vi "First Test.vi"() -> ()   [LabVIEW 2013]
uses:
  source/JKI SM/JKI SM.lvclass
panel:
  out "Macro String":string
  in  "Category":string="UI"
  out "All State Frames":string[](array[string])
  out "State Frames":string[](array[string])
  out "error out 2":errorcluster
  out "Is a JKI State Machine 2":bool
  out "Is a JKI State Machine":bool
  out "error out":errorcluster
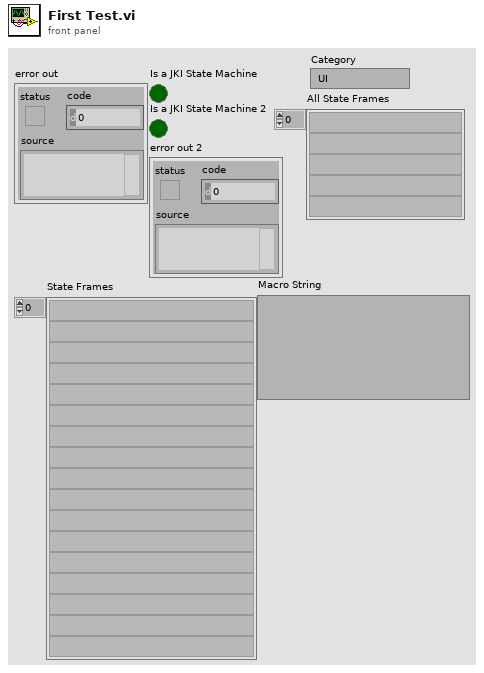
[diagram p1: front panel]
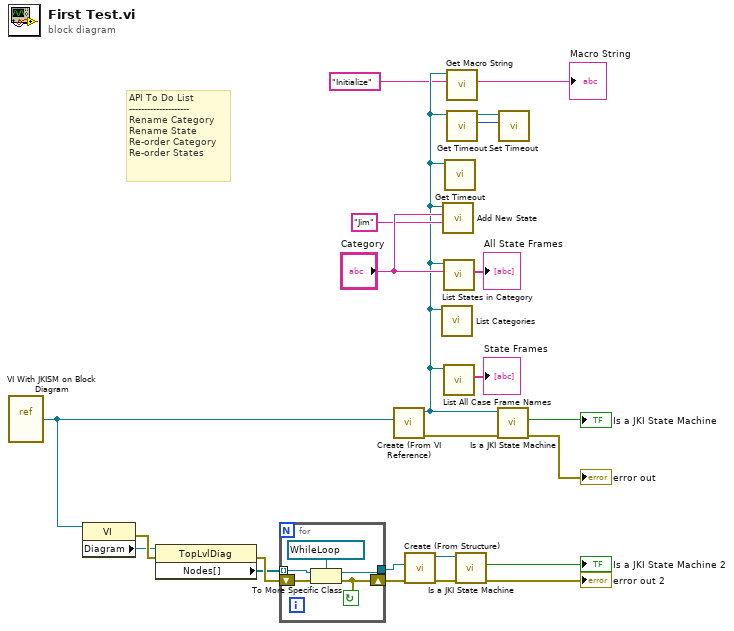
[diagram p0: block diagram]
diagram:
  # "API To Do List\n--------------------\nRename Category\nRename State\nRe-order Category\nRe-order States"
  n1 = vi-ref "VI With JKISM on Block Diagram.vi"() -> (w16:refnum<vi>)
  n2 = property class="VI"(reference=w16) -> (error out=w20:errorcluster, "Diagram"=w17:refnum<vi>)  [unwired: 1 in, 1 out]
  n3 = property class="TopLvlDiag"(reference=w17, error in=w20) -> (error out=w19:errorcluster, "Nodes[]"=w18:refnum<vi>[])  [unwired: 1 out]
  n4 = for {
    tunnel: w18 -> [w27] mode=indexing
    tunnel: [w25] -> w14
    shift-right: [w24] -> w15
    shift-left: w19 -> [w26]
    stop <- w24 continue-if-true
    n5 = To More Specific Class(target class=refnum<vi> refnum ("WLoop Refnum"), reference=w27, error in=w26) -> (specific class reference=w25:refnum<vi>, error out=w24:errorcluster)
  }
  n6 = call "Create (From VI Reference).vi"("VI"=w16) -> ("error out"=w23:errorcluster, "JKI SM out"=w3:refnum<class "JKI SM.lvclass">)  [unwired: 9 in]
  n7 = call "Create (From Structure).vi"("error in (no error)"=w15, "Structure"=w14) -> ("error out"=w13:errorcluster, "JKI SM out"=w12:refnum<class "JKI SM.lvclass">)  [unwired: 8 in]
  n8 = call "List Categories.vi"("JKI SM in"=w3) -> ()  [unwired: 7 in, 4 out]
  n9 = call "Add New State.vi"("State Name"="Jim", "Category (Optional)"="Category", "JKI SM in"=w3) -> ()  [unwired: 7 in, 2 out]
  n10 = call "List States in Category.vi"("Category"="Category", "JKI SM in"=w3) -> ("States"=→"All State Frames":string[])  [unwired: 5 in, 4 out]
  n11 = call "List All Case Frame Names.vi"("JKI SM in"=w3) -> ("All Case Structure Frame Names"=→"State Frames":string[])  [unwired: 8 in, 2 out]
  n12 = call "Get Timeout.vi"("JKI SM in"=w3) -> ()  [unwired: 8 in, 3 out]
  n13 = call "Get Macro String.vi"("Macro Name"="Initialize", "JKI SM in"=w3) -> ("Macro String"=→"Macro String":string)  [unwired: 7 in, 2 out]
  n14 = call "Get Timeout.vi"("JKI SM in"=w3) -> ("Timeout (ms)"=w4:i32, "JKI SM out"=w5:refnum<class "JKI SM.lvclass">)  [unwired: 8 in, 1 out]
  n15 = call "Is a JKI State Machine.vi"("error in (no error)"=w13, "JKI SM in"=w12) -> ("error out"=→"error out 2":errorcluster, "Is a JKI State Machine"=→"Is a JKI State Machine 2":bool)  [unwired: 7 in, 1 out]
  n16 = call "Is a JKI State Machine.vi"("error in (no error)"=w23, "JKI SM in"=w3) -> ("error out"=→"error out":errorcluster, "Is a JKI State Machine"=→"Is a JKI State Machine":bool)  [unwired: 7 in, 1 out]
  n17 = call "Set Timeout.vi"("Timeout (ms)"=w4, "JKI SM in"=w5) -> ()  [unwired: 8 in, 2 out]
